vi "Time Selector.vi"(7 "theme color":u32(colorbox)=2987399, 8 "error in (no error)":errorcluster) -> (0 "error out":errorcluster, 1 "valid":bool, 2 "time stamp":timestamp, 3 "time string":string)   [LabVIEW 2020]
uses:
  <vilib>/Utility/miscctls.llb/LVPoint32TypeDef.ctl
  <vilib>/Utility/miscctls.llb/LVDateTimeRec.ctl
  <vilib>/regexp/Match Regular Expression.xnode
panel:
  out "title month day":string
  out "title year":string
  in  "next month":bool caption="Boolean"
  in  "last month":bool caption="Boolean"
  in  "next year":bool caption="Boolean"
  in  "last year":bool caption="Boolean"
  in  "year input":u16=1906 min=1906 max=2100 step=1
  in  "month select":u16(ring)=1 items=["1月"=1, "2月"=2, "3月"=3, "4月"=4, "5月"=5, "6月"=6, "7月"=7, "8月"=8, "9月"=9, "10月"=10, "11月"=11, "12月"=12]
  out "week header":string[](array[string])
  out "month table":cluster{"selected":bool, "day":string}[][](array[cluster])
  in  "time":string
  in  "cancel":bool caption="Boolean"
  in  "ok":bool caption="Boolean"
  in  "now":bool caption="Boolean"
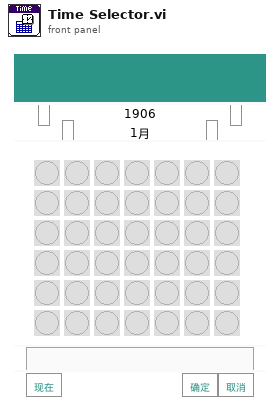
[diagram p1: front panel]
types:
  T1 = typedef "LVPoint32TypeDef.ctl" = cluster{"Horizontal":i32, "Vertical":i32}
  T2 = cluster{"Error":errorcluster, "Exit":bool, "theme color":u32, "time":cluster{"year":u16, "month":u16, "day of month":u16, "hour":u16, "minute":u16, "second":u16, "fractional second":dbl, "day of week":u16}, "month table":cluster{"selected":bool, "day":string}[][], "coords":T1}
  T3 = typedef "LVDateTimeRec.ctl" = cluster{"fractional second":dbl, "second":i32, "minute":i32, "hour":i32, "day of month":i32, "month":i32, "year":i32, "day of week":i32, "day of year":i32, "DST":i32}
  T4 = cluster{"year":u16, "month":u16, "day of month":u16, "hour":u16, "minute":u16, "second":u16, "fractional second":dbl, "day of week":u16}
  T5 = cluster{"year":u16, "month":u16, "day of month":u16}
  T6 = cluster{"year":u16, "month out":u16, "day of month":u16}
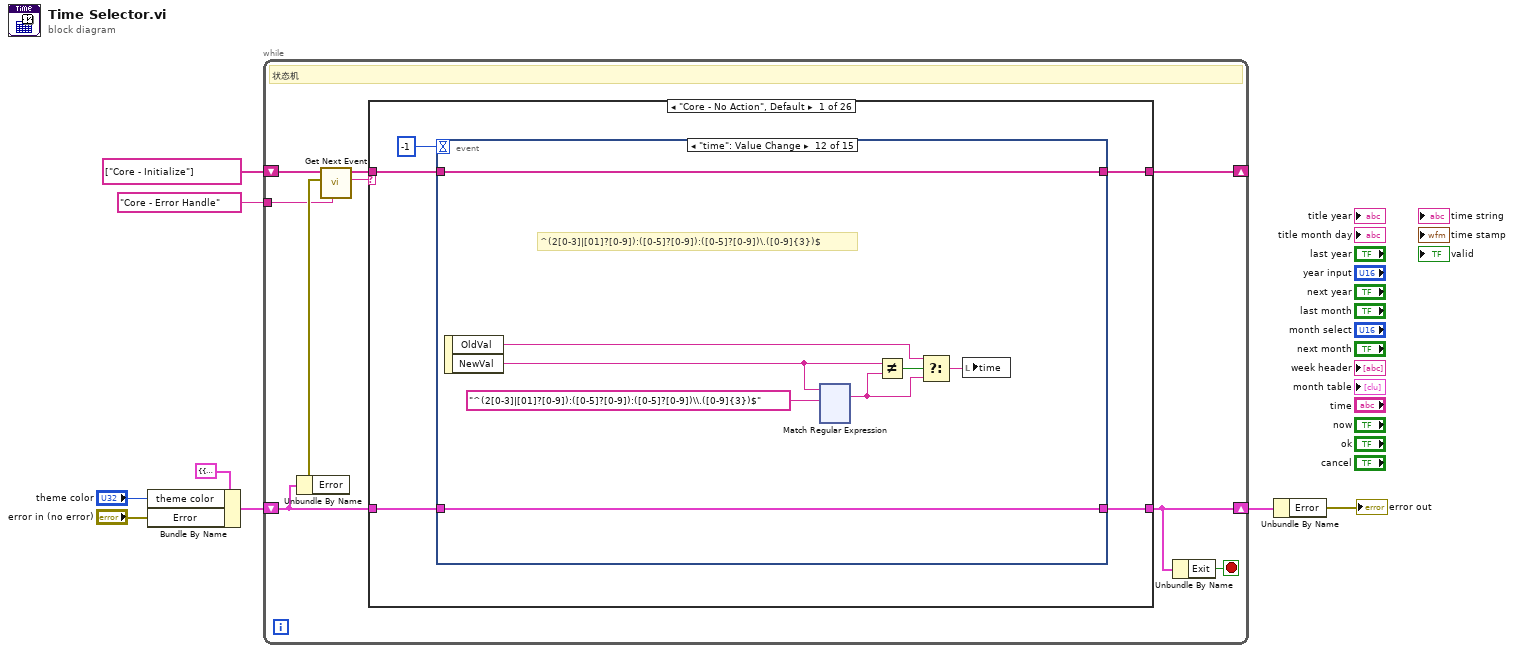
[diagram p0: block diagram]
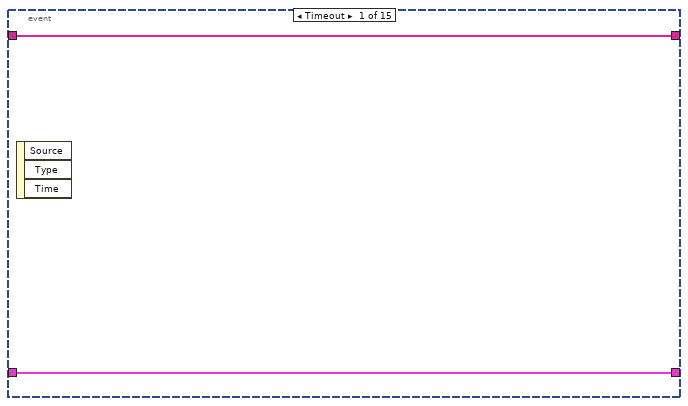
[diagram p2: hidden frame]
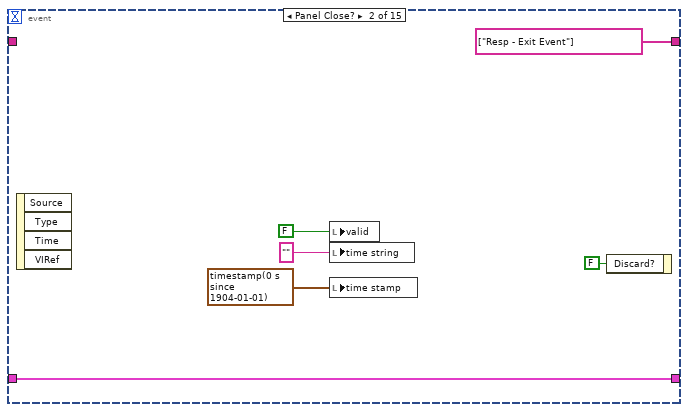
[diagram p3: hidden frame]
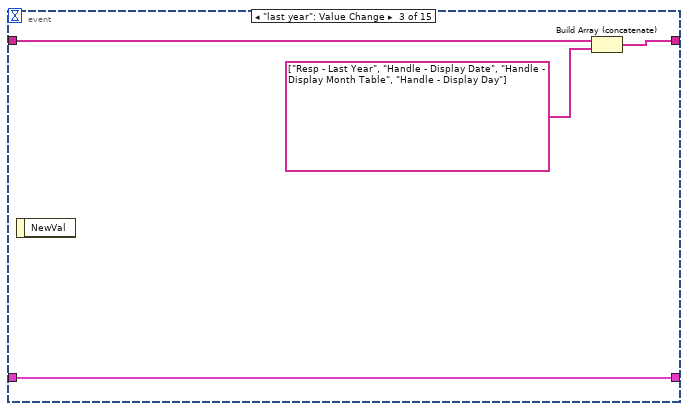
[diagram p4: hidden frame]
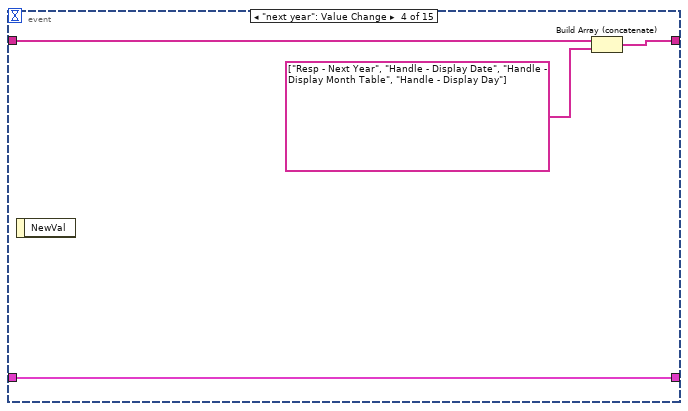
[diagram p5: hidden frame]
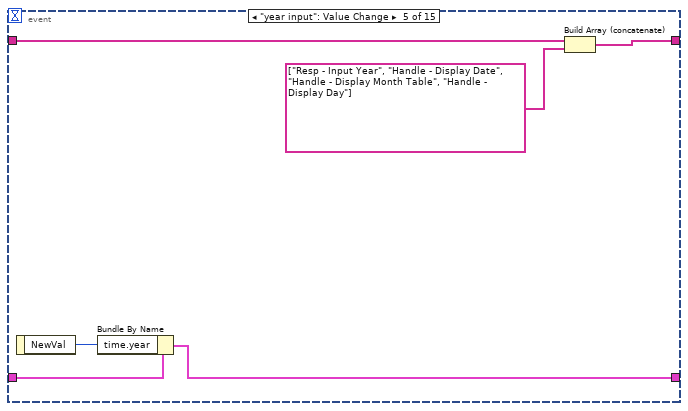
[diagram p6: hidden frame]
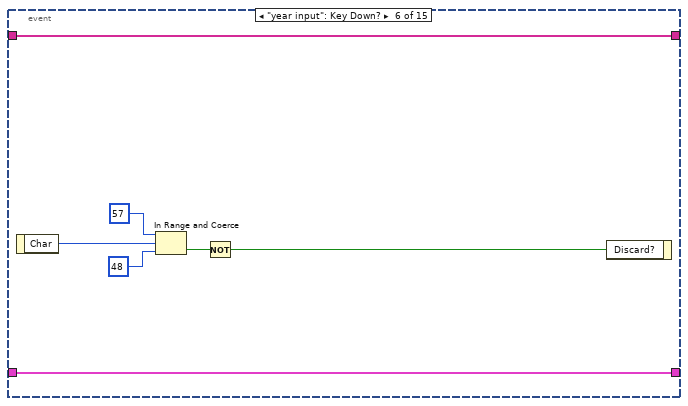
[diagram p7: hidden frame]
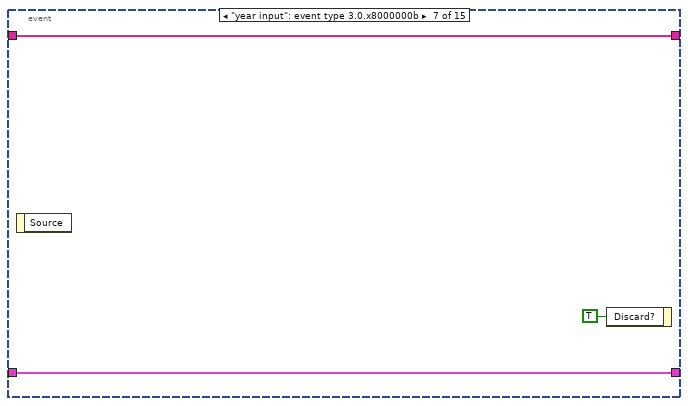
[diagram p8: hidden frame]
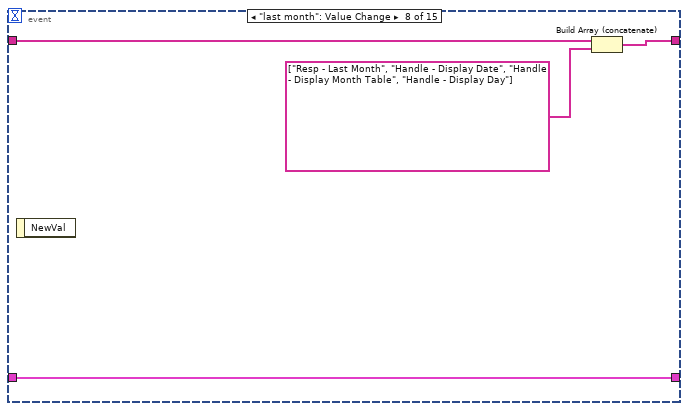
[diagram p9: hidden frame]
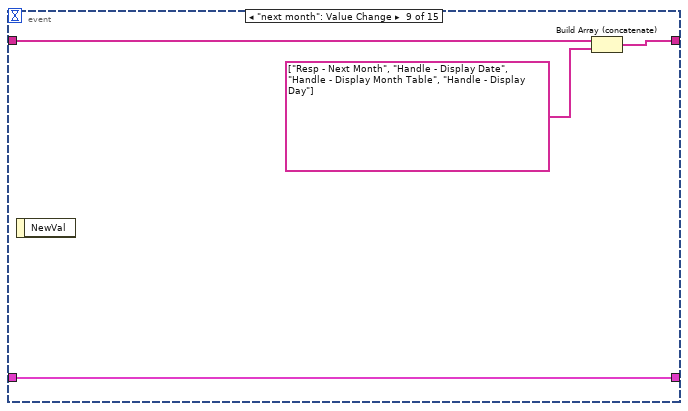
[diagram p10: hidden frame]
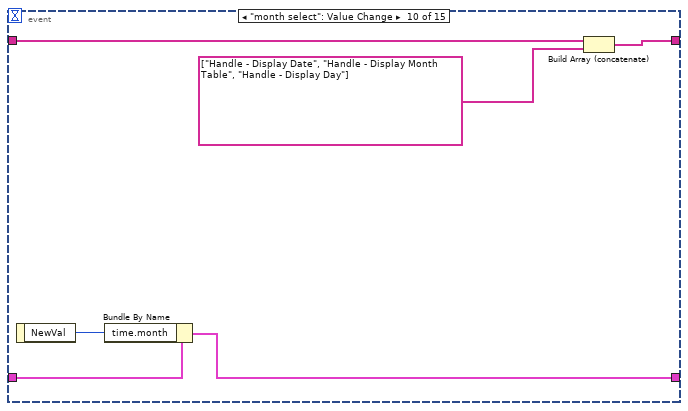
[diagram p11: hidden frame]
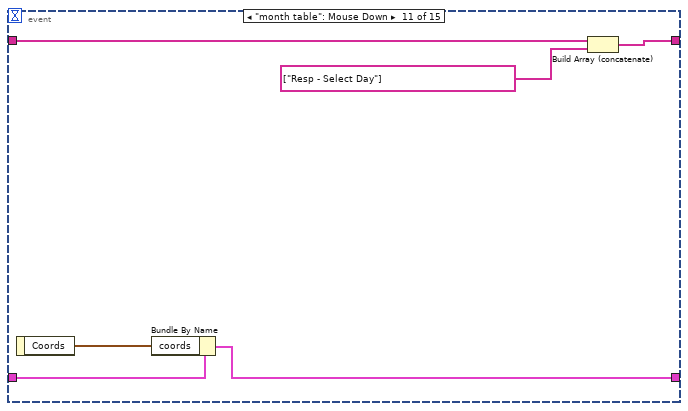
[diagram p12: hidden frame]
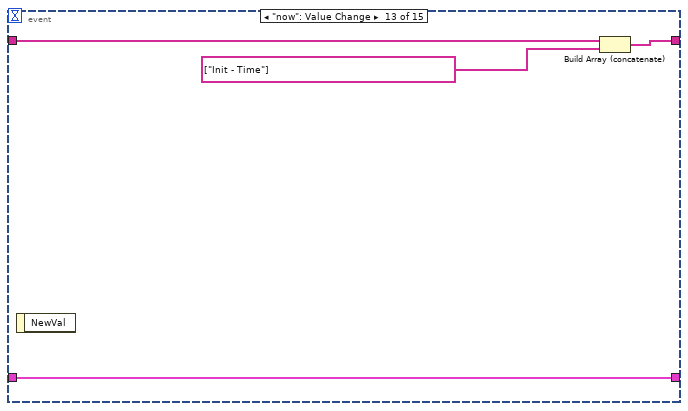
[diagram p13: hidden frame]
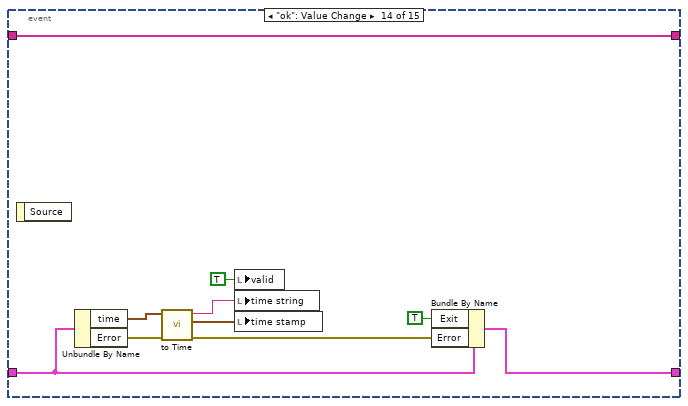
[diagram p14: hidden frame]
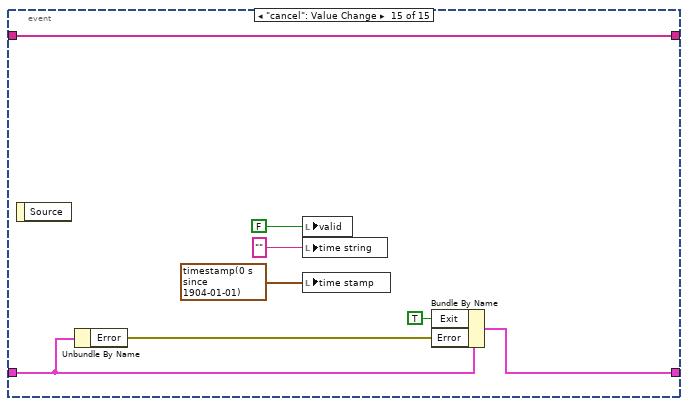
[diagram p15: hidden frame]
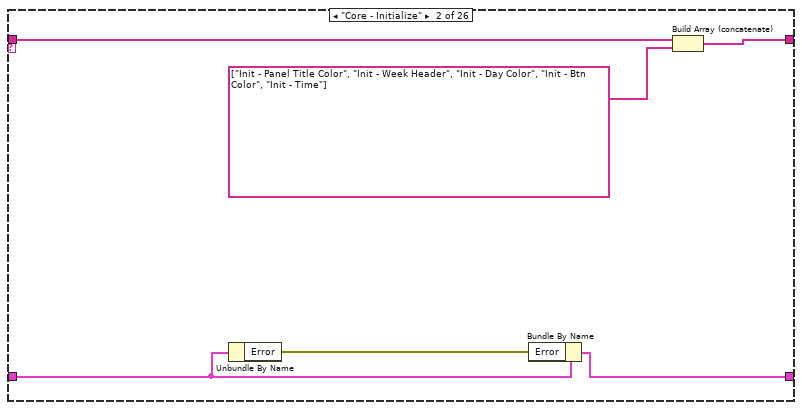
[diagram p16: hidden frame]
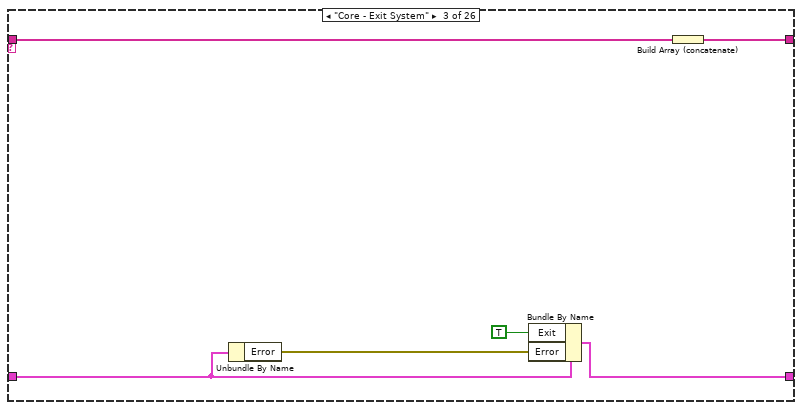
[diagram p17: hidden frame]
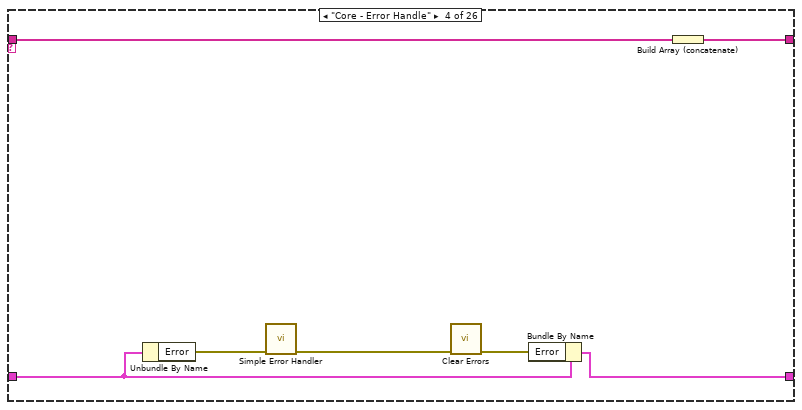
[diagram p18: hidden frame]
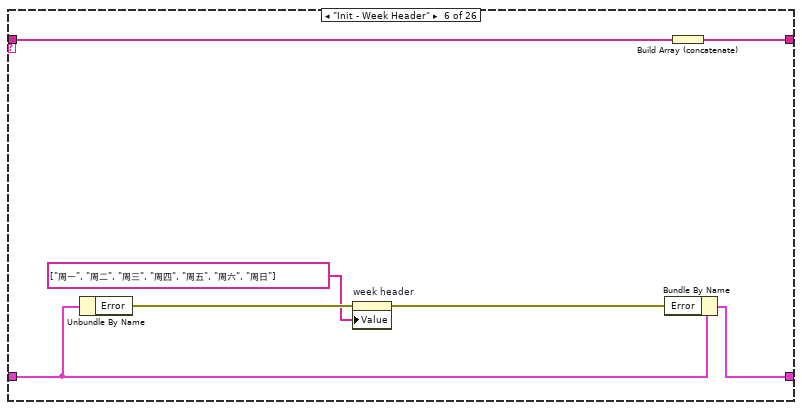
[diagram p20: hidden frame]
diagram:
  n1 = Bundle By Name(cluster=T2 {"Error"={"status"=FALSE, "code"=0, "source"=""}, "Exit"=FALSE, "theme color"=2987399, "time"={"year"=0, "month"=0, "day of month"=0, "hour"=0, "minute"=0, "second"=0, "fractional second"=0.0, "day of week"=0}, "month table"=[], "coords"={"Horizontal"=0, "Vertical"=0}} ("Temp Variable"), "theme color"="theme color", "Error"="error in (no error)") -> (w5:T2)
  n2 = while {
    shift-right: [w12] -> _
    shift-left: string[] ["Core - Initialize"] -> [w15]
    shift-right: [w11] -> w2
    shift-left: w5 -> [w14]
    tunnel: "Core - Error Handle" ("Error Handle") -> [w9]
    stop <- w10 stop-if-true
    # "状态机"
    n3 = Unbundle By Name(w14) -> ("Error"=w13:errorcluster)
    n4 = call <vilib>:"Get Next Event.vi"("Error Handle"=w9, "error in (no error)"=w13, "event queue in"=w15) -> ("next event"=w16:string, "event queue out"=w17:string[])  [unwired: 7 in]
    n5 = case shown="\"Core - No Action\", Default" w16 {
      tunnel: w17 -> [w19 w224 w230 w237 w239 w246 w256 w271 w280 w286 w288 w293 w303 w313 w322 w336 w350 w370 _ w380 w386 w408 w423 w432 w439 w468]
      tunnel: w14 -> [w21 w222 w228 w235 w238 w244 w254 w269 w278 w284 w287 w291 w295 w305 w315 w324 w338 w356 w378 w381 w384 w406 w420 w429 w437 w466]
      tunnel: [w18 w223 w229 w236 w239 w245 w255 w270 w279 w285 w288 w292 w302 w312 w321 w335 w349 w369 w379 w380 w385 w407 w422 w431 w438 w467] -> w12
      tunnel: [w20 w220 w227 w234 w238 w243 w253 w268 w277 w283 w287 w290 w294 w304 w314 w323 w337 w355 w377 w381 w383 w405 w421 w430 w437 w466] -> w11
      frame "Core - No Action", Default {
        n6 = event shown="[11] \"time\": Value Change" {
          selector: _ -> [_ _ _ _ _ _ _ _ _ _ _ _ _ _ _]
          dyn-events: _ -> [_ _ _ _ _ _ _ _ _ _ _ _ _ _ _]
          timeout: -1 -> [_ _ _ _ _ _ _ _ _ _ _ _ _ _ _]
          tunnel: w21 -> [w24 w30 w32 w36 w43 w46 w53 w56 w60 w68 w72 w81 w200 w207 w218]
          tunnel: [w24 w30 w32 w36 w42 w46 w53 w56 w60 w66 w70 w81 w200 w206 w217] -> w20
          tunnel: w19 -> [w23 _ w34 w38 w44 w45 w52 w58 w62 w65 w74 w82 w199 w203 w216]
          tunnel: [w23 string[] ["Resp - Exit Event"] ("event queue out") w33 w37 w40 w45 w52 w57 w61 w64 w73 w82 w198 w203 w216] -> w18
          event Timeout {
            n7 = event-data() -> ()  [unwired: 1 in, 3 out]
          }
          event Panel Close? {
            n8 = event-data() -> ()  [unwired: 1 in, 4 out]
            n9 = local write "valid"(FALSE ("valid")) -> ()
            n10 = local write "time string"("" ("time string")) -> ()
            n11 = local write "time stamp"(timestamp(0 s since 1904-01-01) ("time stamp")) -> ()
            n12 = event-data("Discard?"=FALSE) -> ()  [unwired: 1 in, 1 out]
          }
          event "last year": Value Change {
            n13 = event-data() -> ()  [unwired: 1 in, 1 out]
            n14 = Build Array (concatenate)(w34, string[] ["Resp - Last Year", "Handle - Display Date", "Handle - Display Month Table", "Handle - Display Day"] ("array")) -> (w33:string[])
          }
          event "next year": Value Change {
            (unwired) string[] ["Resp - Next Year", "Handle - Display Date", "Handle - Display Month Table", "Handle - Display Day"] ("array")
            n15 = event-data() -> ()  [unwired: 1 in, 1 out]
            n16 = Build Array (concatenate)(w38, string[] ["Resp - Next Year", "Handle - Display Date", "Handle - Display Month Table", "Handle - Display Day"] ("array")) -> (w37:string[])
          }
          event "year input": Value Change {
            n17 = event-data() -> ("NewVal"=w41:u16)  [unwired: 1 in]
            n18 = Bundle By Name(cluster=w43, "time.year"=w41) -> (w42:T2)
            n19 = Build Array (concatenate)(w44, string[] ["Resp - Input Year", "Handle - Display Date", "Handle - Display Month Table", "Handle - Display Day"] ("array")) -> (w40:string[])
          }
          event "year input": Key Down? {
            n20 = event-data() -> ("Char"=w51:i16)  [unwired: 1 in]
            n21 = In Range and Coerce(upper limit=i16 57, x=w51, lower limit=i16 48) -> (In Range?=w48:bool)  [unwired: 1 out]
            n22 = Not(x=w48) -> (.not. x?=w47:bool)
            n23 = event-data("Discard?"=w47) -> ()  [unwired: 1 in, 1 out]
          }
          event "year input": event type 3.0.x8000000b {
            n24 = event-data() -> ()  [unwired: 1 in, 1 out]
            n25 = event-data("Discard?"=TRUE) -> ()  [unwired: 1 in, 1 out]
          }
          event "last month": Value Change {
            n26 = event-data() -> ()  [unwired: 1 in, 1 out]
            n27 = Build Array (concatenate)(w58, string[] ["Resp - Last Month", "Handle - Display Date", "Handle - Display Month Table", "Handle - Display Day"] ("array")) -> (w57:string[])
          }
          event "next month": Value Change {
            n28 = event-data() -> ()  [unwired: 1 in, 1 out]
            n29 = Build Array (concatenate)(w62, string[] ["Resp - Next Month", "Handle - Display Date", "Handle - Display Month Table", "Handle - Display Day"] ("array")) -> (w61:string[])
          }
          event "month select": Value Change {
            n30 = event-data() -> ("NewVal"=w67:u16)  [unwired: 1 in]
            n31 = Bundle By Name(cluster=w68, "time.month"=w67) -> (w66:T2)
            n32 = Build Array (concatenate)(w65, string[] ["Handle - Display Date", "Handle - Display Month Table", "Handle - Display Day"] ("array")) -> (w64:string[])
          }
          event "month table": Mouse Down {
            n33 = event-data() -> ("Coords"=w71:T1)  [unwired: 1 in]
            n34 = Bundle By Name(cluster=w72, "coords"=w71) -> (w70:T2)
            n35 = Build Array (concatenate)(w74, string[] ["Resp - Select Day"] ("array")) -> (w73:string[])
          }
          event "time": Value Change {
            # "^(2[0-3]|[01]?[0-9]):([0-5]?[0-9]):([0-5]?[0-9])\\.([0-9]{3})$"
            n36 = event-data() -> ("OldVal"=w77:string, "NewVal"=w79:string)  [unwired: 1 in]
            n37 = xnode "Match Regular Expression"("input string"=w79, "regular expression"="^(2[0-3]|[01]?[0-9]):([0-5]?[0-9]):([0-5]?[0-9])\\.([0-9]{3})$") -> ("whole match"=w76:string)  [unwired: 4 in, 4 out]
            n38 = Not Equal?(x=w79, y=w76) -> (x != y?=w78:bool)
            n39 = Select(t=w77, s=w78, f=w76) -> (s? t:f=w75:string)
            n40 = local write "time"(w75) -> ()
          }
          event "now": Value Change {
            n41 = event-data() -> ()  [unwired: 1 in, 1 out]
            n42 = Build Array (concatenate)(w199, string[] ["Init - Time"] ("array")) -> (w198:string[])
          }
          event "ok": Value Change {
            n43 = event-data() -> ()  [unwired: 1 in, 1 out]
            n44 = Unbundle By Name(w207) -> ("time"=w209:T4, "Error"=w210:errorcluster)
            n45 = call "to Time.vi"("error in (no error)"=w210, "time"=w209) -> ("error out"=w208:errorcluster, "time stamp"=w204:timestamp, "time string"=w205:string)  [unwired: 7 in]
            n46 = local write "valid"(TRUE ("valid")) -> ()
            n47 = local write "time string"(w205) -> ()
            n48 = local write "time stamp"(w204) -> ()
            n49 = Bundle By Name(cluster=w207, "Exit"=TRUE, "Error"=w208) -> (w206:T2)
          }
          event "cancel": Value Change {
            n50 = event-data() -> ()  [unwired: 1 in, 1 out]
            n51 = Unbundle By Name(w218) -> ("Error"=w214:errorcluster)
            n52 = local write "valid"(FALSE ("valid")) -> ()
            n53 = local write "time string"("" ("time string")) -> ()
            n54 = local write "time stamp"(timestamp(0 s since 1904-01-01) ("time stamp")) -> ()
            n55 = Bundle By Name(cluster=w218, "Exit"=TRUE, "Error"=w214) -> (w217:T2)
          }
        }
      }
      frame "Core - Initialize" {
        n56 = Unbundle By Name(w222) -> ("Error"=w221:errorcluster)
        n57 = Bundle By Name(cluster=w222, "Error"=w221) -> (w220:T2)
        n58 = Build Array (concatenate)(w224, string[] ["Init - Panel Title Color", "Init - Week Header", "Init - Day Color", "Init - Btn Color", "Init - Time"] ("array")) -> (w223:string[])
      }
      frame "Core - Exit System" {
        n59 = Unbundle By Name(w228) -> ("Error"=w226:errorcluster)
        n60 = Bundle By Name(cluster=w228, "Exit"=TRUE, "Error"=w226) -> (w227:T2)
        n61 = Build Array (concatenate)(w230) -> (w229:string[])
      }
      frame "Core - Error Handle" {
        n62 = Unbundle By Name(w235) -> ("Error"=w233:errorcluster)
        n63 = call <vilib>:"Simple Error Handler.vi"("error in (no error)"=w233) -> ("error out"=w231:errorcluster)  [unwired: 4 in, 4 out]
        n64 = call <vilib>:"Clear Errors.vi"("error in (no error)"=w231) -> ("error out"=w232:errorcluster)  [unwired: 5 in, 1 out]
        n65 = Bundle By Name(cluster=w235, "Error"=w232) -> (w234:T2)
        n66 = Build Array (concatenate)(w237) -> (w236:string[])
      }
      frame "----------------------------------Initialize----------------------------------" {
      }
      frame "Init - Week Header" {
        n67 = Unbundle By Name(w244) -> ("Error"=w242:errorcluster)
        n68 = property on="week header" class="Arr (strict)"(error in=w242, "Value"=string[] ["周一", "周二", "周三", "周四", "周五", "周六", "周日"] ("Array 3")) -> (error out=w241:errorcluster)  [unwired: 1 in, 1 out]
        n69 = Bundle By Name(cluster=w244, "Error"=w241) -> (w243:T2)
        n70 = Build Array (concatenate)(w246) -> (w245:string[])
      }
      frame "Init - Panel Title Color" {
        n71 = control-ref of="Pane"() -> (w252:refnum<vi>)
        n72 = Unbundle By Name(w254) -> ("Error"=w251:errorcluster, "theme color"=w247:u32)
        n73 = property class="Pane"(reference=w252, error in=w251, "PaneColor"=w247) -> (reference out=w249:refnum<vi>, error out=w250:errorcluster)
        n74 = Close Reference(reference=w249, error in (no error)=w250) -> (error out=w248:errorcluster)
        n75 = Bundle By Name(cluster=w254, "Error"=w248) -> (w253:T2)
        n76 = Build Array (concatenate)(w256) -> (w255:string[])
      }
      frame "Init - Day Color" {
        n77 = Unbundle By Name(w269) -> ("Error"=w262:errorcluster, "theme color"=w264:u32)
        n78 = control-ref of="selected"() -> (w261:refnum<vi>)
        n79 = Bundle(cluster=cluster{u32, u32} {2987399, 2987399}, w264, w264) -> (w263:cluster{u32, u32})
        n80 = Replace Array Subset(array=cluster{u32, u32}[] [{16777215, 16777215}, {2987399, 2987399}, {16777216, 16777216}, {16777216, 16777216}] ("Colors [4]"), new element=w263, index=1) -> (w260:cluster{u32, u32}[])
        n81 = property class="Bool (strict)"(reference=w261, error in=w262, "Colors [4]"=w260) -> (reference out=w257:refnum<vi>, error out=w259:errorcluster)
        n82 = Close Reference(reference=w257, error in (no error)=w259) -> (error out=w258:errorcluster)
        n83 = Bundle By Name(cluster=w269, "Error"=w258) -> (w268:T2)
        n84 = Build Array (concatenate)(w271) -> (w270:string[])
      }
      frame "Init - Btn Color" {
        n85 = Unbundle By Name(w278) -> ("Error"=w276:errorcluster, "theme color"=w272:u32)
        n86 = property on="now" class="Bool"(error in=w276, "BoolText.TextColor"=w272) -> (error out=w275:errorcluster)  [unwired: 1 in, 1 out]
        n87 = property on="ok" class="Bool"(error in=w275, "BoolText.TextColor"=w272) -> (error out=w274:errorcluster)  [unwired: 1 in, 1 out]
        n88 = property on="cancel" class="Bool"(error in=w274, "BoolText.TextColor"=w272) -> (error out=w273:errorcluster)  [unwired: 1 in, 1 out]
        n89 = Bundle By Name(cluster=w278, "Error"=w273) -> (w277:T2)
        n90 = Build Array (concatenate)(w280) -> (w279:string[])
      }
      frame "Init - Time" {
        n91 = Unbundle By Name(w284) -> ("Error"=w282:errorcluster)
        n92 = Bundle By Name(cluster=w284, "Error"=w282) -> (w283:T2)
        n93 = Build Array (concatenate)(w286, string[] ["Handle - Get System Time", "Handle - Display Date", "Handle - Display Month Table", "Handle - Display Day", "Handle - Display Time"] ("array")) -> (w285:string[])
      }
      frame "---------------------------------Response---------------------------------" {
      }
      frame "Resp - /* ADD NAME */" {
        n94 = Unbundle By Name(w291) -> ("Error"=w289:errorcluster)
        n95 = Bundle By Name(cluster=w291, "Error"=w289) -> (w290:T2)
        n96 = Build Array (concatenate)(w293) -> (w292:string[])
      }
      frame "Resp - Last Year" {
        n97 = Unbundle By Name(w295) -> ("time.year"=w300:u16, "time.month"=w299:u16, "time.day of month"=w298:u16)
        n98 = Decrement(x=w300) -> (x-1=w296:u16)
        n99 = Bundle(w296, "month"=w299, "day of month"=w298) -> (w297:cluster{u16, "month":u16, "day of month":u16})  [unwired: 1 in]
        n100 = call "Check Leap Year Day.vi"("time"=w297) -> ("day"=w301:u16)  [unwired: 4 in]
        n101 = Bundle By Name(cluster=w295, "time.year"=w296, "time.day of month"=w301) -> (w294:T2)
        n102 = Build Array (concatenate)(w303) -> (w302:string[])
      }
      frame "Resp - Next Year" {
        n103 = Unbundle By Name(w305) -> ("time.year"=w310:u16, "time.month"=w309:u16, "time.day of month"=w308:u16)
        n104 = Increment(x=w310) -> (x+1=w306:u16)
        n105 = Bundle(w306, "month"=w309, "day of month"=w308) -> (w307:cluster{u16, "month":u16, "day of month":u16})  [unwired: 1 in]
        n106 = call "Check Leap Year Day.vi"("time"=w307) -> ("day"=w311:u16)  [unwired: 4 in]
        n107 = Bundle By Name(cluster=w305, "time.year"=w306, "time.day of month"=w311) -> (w304:T2)
        n108 = Build Array (concatenate)(w313) -> (w312:string[])
      }
      frame "Resp - Input Year" {
        n109 = Unbundle By Name(w315) -> ("time.year"=w316:u16, "time.month"=w319:u16, "time.day of month"=w318:u16)
        n110 = Bundle("year"=w316, "month"=w319, "day of month"=w318) -> (w317:T5)  [unwired: 1 in]
        n111 = call "Check Leap Year Day.vi"("time"=w317) -> ("day"=w320:u16)  [unwired: 4 in]
        n112 = Bundle By Name(cluster=w315, "time.day of month"=w320) -> (w314:T2)
        n113 = Build Array (concatenate)(w322) -> (w321:string[])
      }
      frame "Resp - Last Month" {
        n114 = Unbundle By Name(w324) -> ("time.year"=w326:u16, "time.month"=w332:u16, "time.day of month"=w333:u16)
        n115 = call "Last Month.vi"("month in"=w332) -> ("month out"=w330:u16)  [unwired: 4 in]
        n116 = Decrement(x=w326) -> (x-1=w327:u16)
        n117 = Equal?(x=u16 12, y=w330) -> (x = y?=w328:bool)
        n118 = Select(t=w327, s=w328, f=w326) -> (s? t:f=w325:u16)
        n119 = Bundle("year"=w325, "month out"=w330, "day of month"=w333) -> (w331:T6)  [unwired: 1 in]
        n120 = call "Check Leap Year Day.vi"("time"=w331) -> ("day"=w334:u16)  [unwired: 4 in]
        n121 = Bundle By Name(cluster=w324, "time.year"=w325, "time.month"=w330, "time.day of month"=w334) -> (w323:T2)
        n122 = Build Array (concatenate)(w336) -> (w335:string[])
      }
      frame "Resp - Next Month" {
        n123 = Unbundle By Name(w338) -> ("time.year"=w340:u16, "time.month"=w346:u16, "time.day of month"=w347:u16)
        n124 = call "Next Month.vi"("month in"=w346) -> ("month out"=w344:u16)  [unwired: 4 in]
        n125 = Increment(x=w340) -> (x+1=w341:u16)
        n126 = Equal?(x=u16 1, y=w344) -> (x = y?=w342:bool)
        n127 = Select(t=w341, s=w342, f=w340) -> (s? t:f=w339:u16)
        n128 = Bundle("year"=w339, "month out"=w344, "day of month"=w347) -> (w345:T6)  [unwired: 1 in]
        n129 = call "Check Leap Year Day.vi"("time"=w345) -> ("day"=w348:u16)  [unwired: 4 in]
        n130 = Bundle By Name(cluster=w338, "time.year"=w339, "time.month"=w344, "time.day of month"=w348) -> (w337:T2)
        n131 = Build Array (concatenate)(w350) -> (w349:string[])
      }
      frame "Resp - Select Day" {
        n132 = Unbundle By Name(w356) -> ("coords.Vertical"=w366:i32, "coords.Horizontal"=w365:i32)
        n133 = Unbundle By Name(w356) -> ("month table"=w362:cluster{"selected":bool, "day":string}[][])
        n134 = expression code="x-24"(w366) -> (w364:i32)
        n135 = expression code="x-12"(w365) -> (w363:i32)
        n136 = Quotient & Remainder(x=w364, y=30) -> (floor(x/y)=w358:i32)  [unwired: 1 out]
        n137 = Quotient & Remainder(x=w363, y=31) -> (floor(x/y)=w357:i32)  [unwired: 1 out]
        n138 = Index Array(array=w362, index (row)=w358, index (col)=w357) -> (element=w361:cluster{"selected":bool, "day":string})
        n139 = Unbundle By Name(w361) -> ("day"=w360:string)
        n140 = Empty String/Path?(string/path=w360) -> (empty?=w352:bool)
        n141 = Decimal String To Number(string=w360) -> (number=w359:i32)  [unwired: 2 in, 1 out]
        n142 = case shown="False" w352 {
          tunnel: w356 -> [w373 w374]
          tunnel: w359 -> [w372 _]
          tunnel: [w371 w374] -> w355
          frame False {
            n143 = Bundle By Name(cluster=w373, "time.day of month"=w372) -> (w371:T2)
          }
          frame True {
          }
        }
        n144 = Select(t=string[] [] ("day"), s=w352, f=string[] ["Handle - Display Day", "Handle - Display Date"]) -> (s? t:f=w351:string[])
        n145 = Build Array (concatenate)(w370, w351) -> (w369:string[])
      }
      frame "Resp - Exit Event" {
        n146 = Unbundle By Name(w378) -> ("Error"=w376:errorcluster)
        n147 = Bundle By Name(cluster=w378, "Error"=w376) -> (w377:T2)
        n148 = Build Array (concatenate)(string[] ["Core - Exit System"] ("event queue out")) -> (w379:string[])
      }
      frame "----------------------------------Execute-----------------------------------" {
      }
      frame "Handle - /* ADD NAME */" {
        n149 = Unbundle By Name(w384) -> ("Error"=w382:errorcluster)
        n150 = Bundle By Name(cluster=w384, "Error"=w382) -> (w383:T2)
        n151 = Build Array (concatenate)(w386) -> (w385:string[])
      }
      frame "Handle - Get System Time" {
        n152 = Unbundle By Name(w406) -> ("Error"=w403:errorcluster)
        n153 = Get Date/Time In Seconds() -> (seconds since 1Jan1904=w404:timestamp)
        n154 = Seconds To Date/Time(time stamp (now)=w404) -> (date time rec=w402:T3)  [unwired: 1 in]
        n155 = Unbundle By Name(w402) -> ("year"=w395:i32, "month"=w396:i32, "day of month"=w397:i32, "hour"=w398:i32, "minute"=w399:i32, "second"=w400:i32, "fractional second"=w401:dbl, "day of week"=w388:i32)
        n156 = To Unsigned Word Integer(number=w395) -> (unsigned 16bit integer=w394:u16)
        n157 = To Unsigned Word Integer(number=w396) -> (unsigned 16bit integer=w393:u16)
        n158 = To Unsigned Word Integer(number=w397) -> (unsigned 16bit integer=w392:u16)
        n159 = To Unsigned Word Integer(number=w398) -> (unsigned 16bit integer=w391:u16)
        n160 = To Unsigned Word Integer(number=w399) -> (unsigned 16bit integer=w390:u16)
        n161 = To Unsigned Word Integer(number=w400) -> (unsigned 16bit integer=w389:u16)
        n162 = To Unsigned Word Integer(number=w388) -> (unsigned 16bit integer=w387:u16)
        n163 = Bundle By Name(cluster=w406, "time.year"=w394, "time.month"=w393, "time.day of month"=w392, "time.hour"=w391, "time.minute"=w390, "time.second"=w389, "time.fractional second"=w401, "time.day of week"=w387, "Error"=w403) -> (w405:T2)
        n164 = Build Array (concatenate)(w408) -> (w407:string[])
      }
      frame "Handle - Display Date" {
        n165 = Unbundle By Name(w420) -> ("time.year"=w411:u16, "time.month"=w409:u16, "Error"=w412:errorcluster, "time.day of week"=w418:u16, "time.month"=w416:u16, "time.day of month"=w415:u16)
        n166 = Number To Decimal String(number=w411) -> (decimal integer string=w410:string)  [unwired: 1 in]
        n167 = local write "title year"(w410) -> ()
        n168 = local write "year input"(w411) -> ()
        n169 = local write "month select"(w409) -> ()
        n170 = call "to CH Day of Week.vi"("day of week"=w418) -> ("ch day of week"=w419:string)  [unwired: 4 in]
        n171 = Format Into String(format string="%s，%d月%d日", error in=w412, w419, w416, w415) -> (resulting string=w413:string, error out=w414:errorcluster)  [unwired: 1 in]
        n172 = local write "title month day"(w413) -> ()
        n173 = Bundle By Name(cluster=w420, "Error"=w414) -> (w421:T2)
        n174 = Build Array (concatenate)(w423) -> (w422:string[])
      }
      frame "Handle - Display Month Table" {
        n175 = Unbundle By Name(w429) -> ("time.year"=w427:u16, "time.month"=w428:u16, "Error"=w425:errorcluster)
        n176 = Bundle("year"=w427, "month"=w428) -> (w426:cluster{"year":u16, "month":u16})  [unwired: 1 in]
        n177 = call "Cal Month Table.vi"("date"=w426) -> ("month table"=w424:cluster{"selected":bool, "day":string}[][])  [unwired: 4 in]
        n178 = local write "month table"(w424) -> ()
        n179 = Bundle By Name(cluster=w429, "month table"=w424, "Error"=w425) -> (w430:T2)
        n180 = Build Array (concatenate)(w432) -> (w431:string[])
      }
      frame "Handle - Display Day" {
        n181 = Unbundle By Name(w437) -> ("month table"=w436:cluster{"selected":bool, "day":string}[][], "time.day of month"=w435:u16)
        n182 = Number To Decimal String(number=w435) -> (decimal integer string=w434:string)  [unwired: 1 in]
        n183 = for {
          tunnel: w436 -> [w442] mode=indexing
          tunnel: w434 -> [w441]
          tunnel: [w440] -> w433 mode=indexing
          n184 = for {
            tunnel: w442 -> [w446] mode=indexing
            tunnel: w441 -> [w447]
            tunnel: [w445] -> w440 mode=indexing
            n185 = Unbundle(w446) -> ("day"=w444:string)  [unwired: 1 out]
            n186 = Equal?(x=w444, y=w447) -> (x = y?=w443:bool)
            n187 = Bundle(cluster=w446, "selected"=w443, "day"=w444) -> (w445:cluster{"selected":bool, "day":string})
          }
        }
        n188 = local write "month table"(w433) -> ()
        n189 = Build Array (concatenate)(w439) -> (w438:string[])
      }
      frame "Handle - Display Time" {
        n190 = Unbundle By Name(w466) -> ("time.year"=w454:u16, "time.month"=w453:u16, "time.day of month"=w452:u16, "time.hour"=w461:u16, "time.minute"=w464:u16, "time.second"=w463:u16, "time.fractional second"=w462:dbl)
        n191 = To Long Integer(number=w454) -> (32bit integer=w450:i32)
        n192 = To Long Integer(number=w453) -> (32bit integer=w449:i32)
        n193 = To Long Integer(number=w452) -> (32bit integer=w448:i32)
        n194 = To Long Integer(number=w461) -> (32bit integer=w460:i32)
        n195 = To Long Integer(number=w464) -> (32bit integer=w459:i32)
        n196 = To Long Integer(number=w463) -> (32bit integer=w458:i32)
        n197 = Bundle By Name(cluster=T3 {"fractional second"=0.0, "second"=0, "minute"=0, "hour"=0, "day of month"=0, "month"=0, "year"=0, "day of week"=0, "day of year"=0, "DST"=0} ("date time rec"), "year"=w450, "month"=w449, "day of month"=w448, "hour"=w460, "minute"=w459, "second"=w458, "fractional second"=w462) -> (w451:T3)
        n198 = Date/Time To Seconds(2:w451) -> (0:w457:timestamp)  [unwired: 1 in]
        n199 = Format Date/Time String(time format string (%c)="%H:%M:%S%3u" ("format string"), seconds (now)=w457) -> (date/time string=w455:string)  [unwired: 1 in]
        n200 = local write "time"(w455) -> ()
        n201 = Build Array (concatenate)(w468) -> (w467:string[])
      }
    }
    n202 = Unbundle By Name(w11) -> ("Exit"=w10:bool)
  }
  n203 = Unbundle By Name(w2) -> ("Error"=→"error out":errorcluster)
